vi "Configure_TW.vi"() -> (1 "changed?":bool, 2 "Property":string[](array[string]), 3 "Thing":string)   [LabVIEW 2019]
uses:
  <vilib>/Utility/miscctls.llb/LVRowAndColumnUnsignedTypeDef.ctl
panel:
  in  "Properties":i32(listbox)
  in  "Cancel":bool
  in  "OK":bool
  in  "Thing":u16(ring) items=["AR_Project", "Day1"]
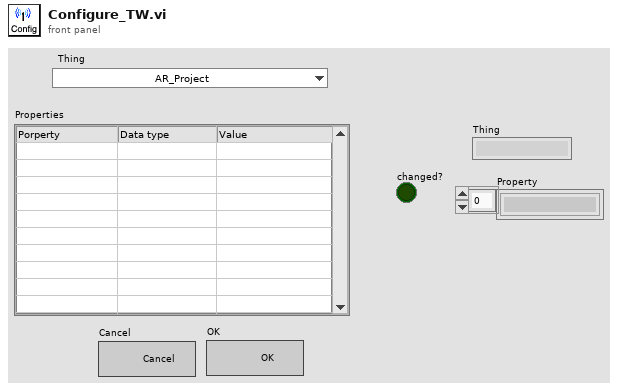
[diagram p1: front panel]
types:
  T1 = typedef "LVRowAndColumnUnsignedTypeDef.ctl" = cluster{"Row":u32, "Column":u32}
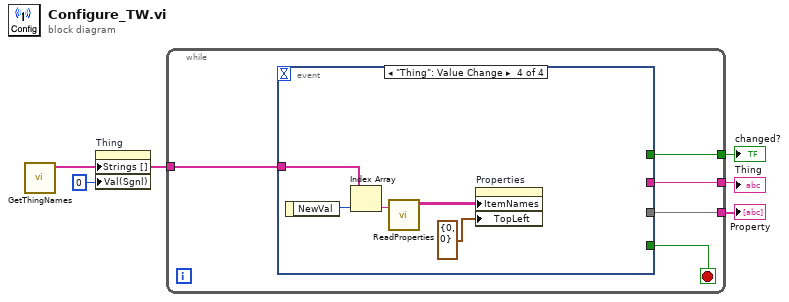
[diagram p0: block diagram]
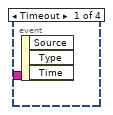
[diagram p2: hidden frame]
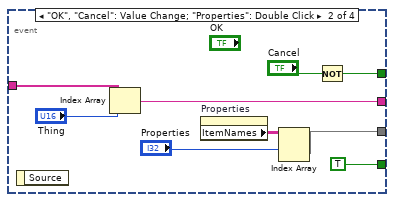
[diagram p3: hidden frame]
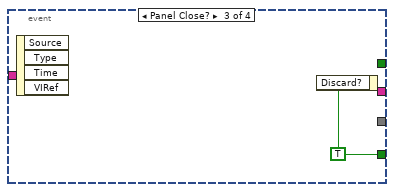
[diagram p4: hidden frame]
diagram:
  n1 = call "GetThingNames.vi"() -> ("Things"=w3:string[])  [unwired: 10 in, 1 out]
  n2 = property on="Thing" class="Ring (strict)"("Strings []"=w3, "Val(Sgnl)"=u16 0 ("Value (Signaling)")) -> ()  [unwired: 2 in, 2 out]
  n3 = while {
    tunnel: [w10] -> w4
    tunnel: w3 -> [w8]
    tunnel: [w7] -> w2
    tunnel: [w6] -> w1
    stop <- w9 stop-if-true
    n4 = event shown="[3] \"Thing\": Value Change" {
      selector: _ -> [_ _ _ _]
      dyn-events: _ -> [_ _ _ _]
      timeout: _ -> [_ _ _ _]
      tunnel: [_ w11 _ _] -> w10
      tunnel: [_ TRUE w20 _] -> w9
      tunnel: w8 -> [_ w18 _ w24]
      tunnel: [_ w16 _ _] -> w7
      tunnel: [_ w13 _ _] -> w6
      event Timeout {
        n5 = event-data() -> ()  [unwired: 1 in, 3 out]
      }
      event "OK", "Cancel": Value Change; "Properties": Double Click {
        n6 = event-data() -> ()  [unwired: 1 in, 1 out]
        n7 = Index Array(array=w18, index="Thing") -> (element=w16:string)
        n8 = property on="Properties" class="MCListbox (strict)"() -> ("ItemNames"=w15:string[][])  [unwired: 2 in, 2 out]
        n9 = Index Array(array=w15, index (row)="Properties") -> (element=w13:string[])  [unwired: 1 in]
        n10 = Not(x="Cancel") -> (.not. x?=w11:bool)
      }
      event Panel Close? {
        w20 = TRUE
        n11 = event-data() -> ()  [unwired: 1 in, 4 out]
        n12 = event-data("Discard?"=w20) -> ()  [unwired: 1 in, 1 out]
      }
      event "Thing": Value Change {
        n13 = event-data() -> ("NewVal"=w25:u16)  [unwired: 1 in]
        n14 = Index Array(array=w24, index=w25) -> (element=w23:string)
        n15 = call "ReadProperties.vi"("Thing"=w23) -> ("All"=w22:string[][])  [unwired: 10 in]
        n16 = property on="Properties" class="MCListbox (strict)"("ItemNames"=w22, "TopLeft"=T1 {"Row"=0, "Column"=0} ("Top Left Visible Cell")) -> ()  [unwired: 2 in, 2 out]
      }
    }
  }
  "changed?" <- w4
  "Thing" <- w2
  "Property" <- w1
